vi "station3_bit to array.vi"(8 "error in (no error)":errorcluster, 11 "ST3_Controls_from_PLC":i64[](array[numeric])=[0, 0, 0, 0, 0]) -> (0 "error out":errorcluster, 2 "3 on state":i32[](array[numeric]), 3 "3 result array":bool[](array[boolean]))   [LabVIEW 2017]
panel:
  out "fpl st3":bool
  out "driver st3":bool
  out "LB st3":bool
  out "cycle rslt 3":bool
  out "HB st3":bool
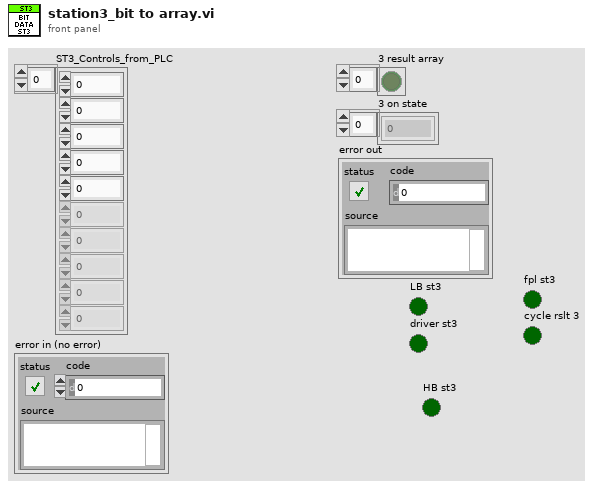
[diagram p1: front panel]
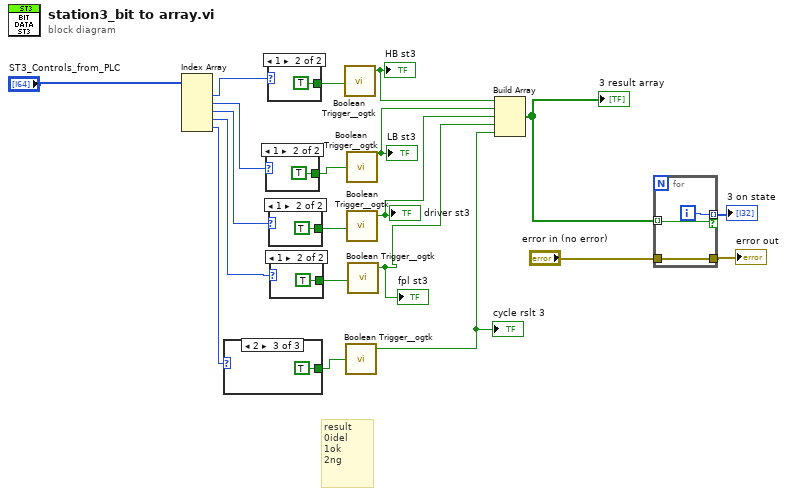
[diagram p0: block diagram]
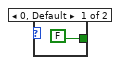
[diagram p2: hidden frame]
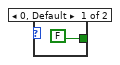
[diagram p3: hidden frame]
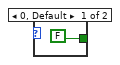
[diagram p4: hidden frame]
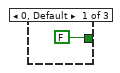
[diagram p5: hidden frame]
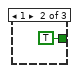
[diagram p6: hidden frame]
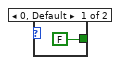
[diagram p7: hidden frame]
diagram:
  # "result\n0idel\n1ok\n2ng"
  n1 = Index Array(array="ST3_Controls_from_PLC") -> (element #1=w20:i64, element #2=w4:i64, element #3=w3:i64, element #4=w2:i64, element #5=w1:i64)  [unwired: 5 in]
  n2 = case shown="2" w1 {
    tunnel: [FALSE TRUE TRUE] -> w19
    frame 0, Default {
    }
    frame 1 {
    }
    frame 2 {
    }
  }
  n3 = case shown="1" w4 {
    tunnel: [FALSE TRUE] -> w10
    frame 0, Default {
    }
    frame 1 {
    }
  }
  n4 = case shown="1" w20 {
    tunnel: [FALSE TRUE] -> w18
    frame 0, Default {
    }
    frame 1 {
    }
  }
  n5 = case shown="1" w3 {
    tunnel: [FALSE TRUE] -> w11
    frame 0, Default {
    }
    frame 1 {
    }
  }
  n6 = case shown="1" w2 {
    tunnel: [FALSE TRUE] -> w9
    frame 0, Default {
    }
    frame 1 {
    }
  }
  n7 = call <userlib>:"Boolean Trigger__ogtk.vi"("Boolean Input"=w18) -> ("Rising Edge"=w16:bool)  [unwired: 1 in, 1 out]
  "HB st3" <- w16
  n8 = call <userlib>:"Boolean Trigger__ogtk.vi"("Boolean Input"=w19) -> ("Rising Edge"=w8:bool)  [unwired: 1 in, 1 out]
  "cycle rslt 3" <- w8
  n9 = call <userlib>:"Boolean Trigger__ogtk.vi"("Boolean Input"=w10) -> ("Rising Edge"=w7:bool)  [unwired: 1 in, 1 out]
  "LB st3" <- w7
  n10 = call <userlib>:"Boolean Trigger__ogtk.vi"("Boolean Input"=w11) -> ("Rising Edge"=w6:bool)  [unwired: 1 in, 1 out]
  "driver st3" <- w6
  n11 = call <userlib>:"Boolean Trigger__ogtk.vi"("Boolean Input"=w9) -> ("Rising Edge"=w5:bool)  [unwired: 1 in, 1 out]
  "fpl st3" <- w5
  n12 = Build Array(w16, w7, w6, w5, w8) -> (w15:bool[])
  "3 result array" <- w15
  n13 = for {
    tunnel: [w34] -> w14 mode=indexing if=w32
    tunnel: "error in (no error)" -> [w33]
    tunnel: [w33] -> w13
    tunnel: w15 -> [w32] mode=indexing
    i -> [w34]
  }
  "3 on state" <- w14
  "error out" <- w13
